vi "serpenbot_DDPG_control.vi"() -> ()   [LabVIEW 2019]
uses:
  <vilib>/Analysis/Matrix/Datatypes/RealMatrix.ctl
  <vilib>/Analysis/Matrix/NI_Matrix.lvlib
  <vilib>/Analysis/NI_AALBase.lvlib
  <vilib>/Analysis/baseanly.llb/Real A x B.vi
  <vilib>/Analysis/Matrix/Numeric/Conversions/Array To Matrix - RA.vi
  <vilib>/Analysis/Matrix/Numeric/Subtract/Subtract - RM,RM.vi
  <vilib>/Analysis/NI_AALPro.lvlib
  <vilib>/Analysis/_algsub.llb/Real PseudoInverse Matrix.vi
panel:
  out "error out Y":errorcluster
  out "error out X":errorcluster
  in  "goal y":dbl
  in  "goal x":dbl
  out "control_loop_time":u32
  in  "stop":bool
  in  "Logging":bool caption="Enable"
  out "laser control value":dbl[](array[numeric])
  in  "k":T1
  in  "Diode Current\nSetting":dbl=3.0
  in  "Laser Repetition\nFrequency":i32=50000
  in  "VISA resource name":refnum<visa-resource-name>="COM14"
  in  "baud rate (9600)":u32=9600
  out "error out":errorcluster
  out "Identification system 1":string
  out "Conn. axes system 1":string[](array[string])
  out "Identification system 2":string
  out "Conn. axes system  2":string[](array[string])
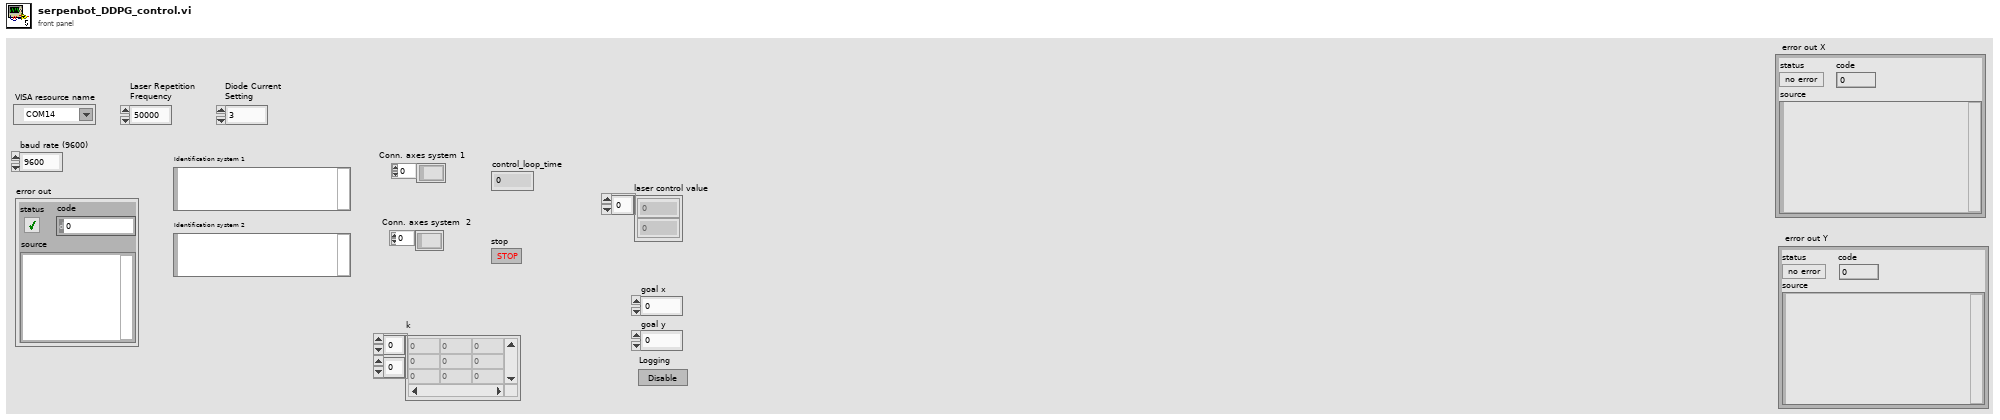
[diagram p1: front panel]
types:
  T1 = typedef "NI_Matrix.lvlib/RealMatrix.ctl" = dbl[][]
  T2 = cluster{"RS232 settings":cluster{"Portnumber":i32, "Baudrate":u16}, "USB settings":cluster{"S/N":string, "USB Search?":bool}, "TCP/IP settings":cluster{"Host address/name":string, "Port":i32, "Board":i32, "TCP/IP Search?":bool}}
  T3 = cluster{"Check FRF?":bool, "Referencing mode":enum16{"FRF (-> FNL)", "FRF", "FNL", "FPL", "RON OFF"}[]}
  T4 = cluster{"Force?":bool, "Dialog?":bool, "Stages":string[]}
  T5 = cluster{"Position":cluster{"x":sgl, "y":sgl}, "Angle":sgl, "Scale":sgl, "Score":sgl, "Bounding Box":cluster{"x":sgl, "y":sgl}[]}[]
  T6 = cluster{"[0]":cluster{"Position":cluster{"x":sgl, "y":sgl}, "Angle":sgl, "Scale":sgl, "Score":sgl, "Bounding Box":cluster{"x":sgl, "y":sgl}[]}, "[1]":cluster{"Position":cluster{"x":sgl, "y":sgl}, "Angle":sgl, "Scale":sgl, "Score":sgl, "Bounding Box":cluster{"x":sgl, "y":sgl}[]}, "[2]":cluster{"Position":cluster{"x":sgl, "y":sgl}, "Angle":sgl, "Scale":sgl, "Score":sgl, "Bounding Box":cluster{"x":sgl, "y":sgl}[]}, "[3]":cluster{"Position":cluster{"x":sgl, "y":sgl}, "Angle":sgl, "Scale":sgl, "Score":sgl, "Bounding Box":cluster{"x":sgl, "y":sgl}[]}, "[4]":cluster{"Position":cluster{"x":sgl, "y":sgl}, "Angle":sgl, "Scale":sgl, "Score":sgl, "Bounding Box":cluster{"x":sgl, "y":sgl}[]}, "[5]":cluster{"Position":cluster{"x":sgl, "y":sgl}, "Angle":sgl, "Scale":sgl, "Score":sgl, "Bounding Box":cluster{"x":sgl, "y":sgl}[]}, "[6]":cluster{"Position":cluster{"x":sgl, "y":sgl}, "Angle":sgl, "Scale":sgl, "Score":sgl, "Bounding Box":cluster{"x":sgl, "y":sgl}[]}, "[7]":cluster{"Position":cluster{"x":sgl, "y":sgl}, "Angle":sgl, "Scale":sgl, "Score":sgl, "Bounding Box":cluster{"x":sgl, "y":sgl}[]}, "[8]":cluster{"Position":cluster{"x":sgl, "y":sgl}, "Angle":sgl, "Scale":sgl, "Score":sgl, "Bounding Box":cluster{"x":sgl, "y":sgl}[]}}
  T7 = cluster{"Position":cluster{"x":sgl, "y":sgl}, "Angle":sgl, "Scale":sgl, "Score":sgl, "Bounding Box":cluster{"x":sgl, "y":sgl}[]}
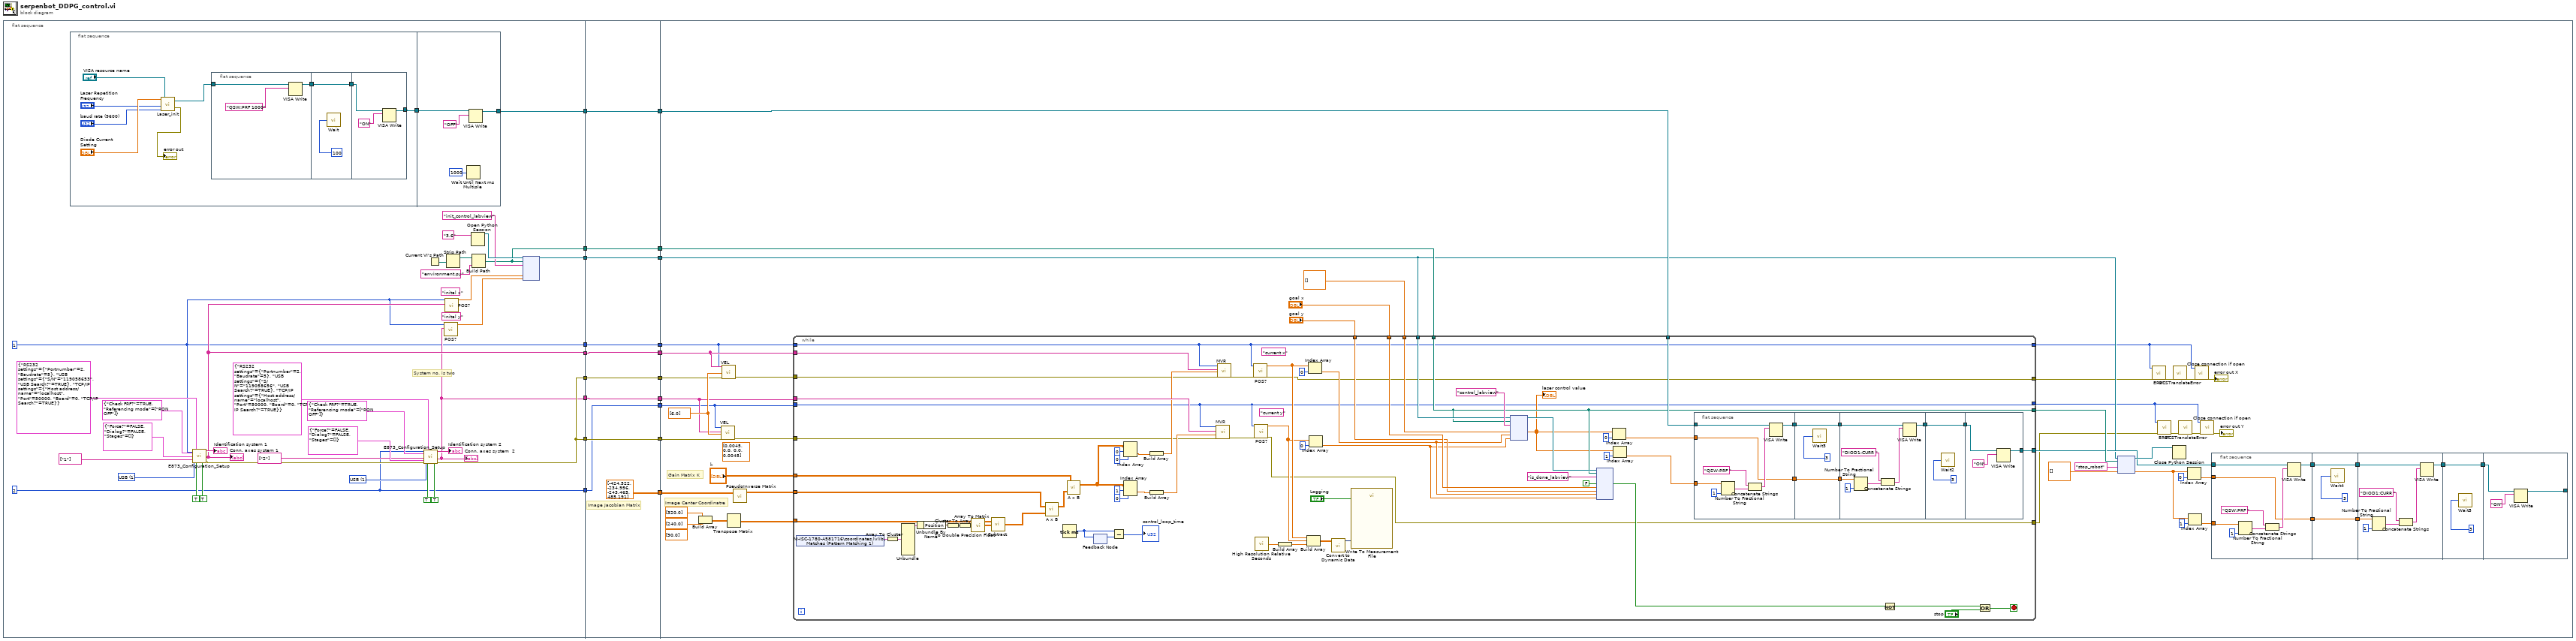
[diagram p0: block diagram]
diagram:
  n1 = flat-sequence {
    tunnel: [w52] -> w19
    tunnel: [w22] -> w18
    tunnel: [w24] -> w17
    tunnel: [w33] -> w16
    tunnel: [w23] -> w15
    tunnel: [w34] -> w14
    tunnel: [w33] -> w13
    tunnel: [w26] -> w12
    tunnel: [w25] -> w11
    tunnel: w19 -> [w84]
    tunnel: [w84] -> w10
    tunnel: w18 -> [w83]
    tunnel: w17 -> [w82]
    tunnel: w16 -> [w81]
    tunnel: w15 -> [w80]
    tunnel: w14 -> [w78]
    tunnel: [w83] -> w9
    tunnel: [w82] -> w8
    tunnel: [w81] -> w7
    tunnel: [w80] -> w6
    tunnel: w13 -> [w79]
    tunnel: [w79] -> w5
    tunnel: [w78] -> w4
    tunnel: [T1 [[-424.522, -234.956], [-243.465, 485.191]] ("J_init 2")] -> w3
    tunnel: w12 -> [w76]
    tunnel: w11 -> [w75]
    tunnel: [w76] -> w2
    tunnel: [w75] -> w1
    tunnel: w10 -> [w132]
    tunnel: w9 -> [w117]
    tunnel: w8 -> [w124]
    tunnel: w7 -> [w127]
    tunnel: w6 -> [w122]
    tunnel: w5 -> [w126]
    tunnel: w4 -> [w116]
    tunnel: w3 -> [w125]
    tunnel: w2 -> [w115]
    tunnel: w1 -> [w98]
    frame #0 {
      (unwired) "inital y"
      (unwired) "inital x"
      w37 = u16 1 items=["RS232", "USB", "TCP/IP"] ("Interface")
      w40 = u16 1 items=["RS232", "USB", "TCP/IP"] ("Interface")
      w34 = 2 ("System no.")
      w22 = 1 ("System no.")
      # "System no. is two"
      n2 = flat-sequence {
        tunnel: [w54] -> w53
        tunnel: w53 -> [w72]
        tunnel: [w71] -> w52
        frame #0 {
          n3 = call "Laser_init.vi"("baud rate (9600)"="baud rate (9600)", "Laser Repetition\nFrequency"="Laser Repetition\nFrequency", "VISA resource name"="VISA resource name", "Diode Current\nSetting"="Diode Current\nSetting") -> ("error out"=→"error out":errorcluster, "VISA Refnum out"=w55:refnum<visa-resource-name>)
          n4 = flat-sequence {
            tunnel: w55 -> [w65]
            tunnel: [w64] -> w62
            tunnel: w62 -> [w67]
            tunnel: [w67] -> w61
            tunnel: w61 -> [w68]
            tunnel: [w69] -> w54
            frame #0 {
              n5 = VISA Write(VISA resource name=w65, write buffer="QSW:PRF 1000" ("string")) -> (VISA resource name out=w64:refnum<visa-resource-name>)  [unwired: 1 in, 2 out]
            }
            frame #1 {
              n6 = call "Wait"("Count(mSec)"=u32 100) -> ()  [unwired: 1 out]
            }
            frame #2 {
              n7 = VISA Write(VISA resource name=w68, write buffer="ON") -> (VISA resource name out=w69:refnum<visa-resource-name>)  [unwired: 1 in, 2 out]
            }
          }
        }
        frame #1 {
          n8 = Wait Until Next ms Multiple(millisecond multiple=u32 1000) -> ()  [unwired: 1 out]
          n9 = VISA Write(VISA resource name=w72, write buffer="OFF") -> (VISA resource name out=w71:refnum<visa-resource-name>)  [unwired: 1 in, 2 out]
        }
      }
      n10 = call "E873_Configuration_Setup.vi"("System no."=w22, "Referencing"=T3 {"Check FRF?"=TRUE, "Referencing mode"=[enum."RON OFF"]}, "Interface"=w40, "All axes?"=TRUE, "Axes to move"=string[] ["1"], "Interface settings"=T2 {"RS232 settings"={"Portnumber"=2, "Baudrate"=5}, "USB settings"={"S/N"="119058653", "USB Search?"=TRUE}, "TCP/IP settings"={"Host address/name"="localhost", "Port"=50000, "Board"=0, "TCP/IP Search?"=TRUE}}, "Stage selection"=T4 {"Force?"=FALSE, "Dialog?"=FALSE, "Stages"=[]}, "Switch servo on?"=TRUE ("Use dialog to define\nconnected stages?")) -> ("Identification"=→"Identification system 1":string, "Conn. \nAxes"=w24:string[], "error out"=w49:errorcluster)  [unwired: 4 in, 5 out]
      "Conn. axes system 1" <- w24
      n11 = call "E873_Configuration_Setup.vi"("System no."=w34, "Referencing"=T3 {"Check FRF?"=TRUE, "Referencing mode"=[enum."RON OFF"]}, "Interface"=w37, "All axes?"=TRUE, "Axes to move"=string[] ["2"], "error in"=w49, "Interface settings"=T2 {"RS232 settings"={"Portnumber"=2, "Baudrate"=5}, "USB settings"={"S/N"="119058656", "USB Search?"=TRUE}, "TCP/IP settings"={"Host address/name"="localhost", "Port"=50000, "Board"=0, "TCP/IP Search?"=TRUE}}, "Stage selection"=T4 {"Force?"=FALSE, "Dialog?"=FALSE, "Stages"=[]}, "Switch servo on?"=TRUE ("Use dialog to define\nconnected stages?")) -> ("Identification"=→"Identification system 2":string, "Conn. \nAxes"=w23:string[], "error out"=w33:errorcluster)  [unwired: 3 in, 5 out]
      "Conn. axes system  2" <- w23
      n12 = Current VI's Path() -> (path=w32:path)
      n13 = call "POS?.vi"("System no."=w22, "Axes to query"=w23) -> ("Position"=w20:dbl[])  [unwired: 3 in, 14 out]
      n14 = call "POS?.vi"("System no."=w22, "Axes to query"=w24) -> ("Position"=w21:dbl[])  [unwired: 3 in, 14 out]
      n15 = Strip Path(path=w32) -> (stripped path=w31:path)  [unwired: 1 out]
      n16 = Open Python Session(python version="3.6" ("Python version")) -> (session out=w28:refnum<k35>)  [unwired: 2 in, 1 out]
      n17 = Build Path(base path=w31, name or relative path="environment.py") -> (appended path=w26:path)
      n18 = node(w28, w26, "init_control_labview" ("function name"), w21, w20) -> (w25:refnum<k35>)  [unwired: 5 in, 3 out]
    }
    frame #1 {
      # "Image Jacobian Matrix"
    }
    frame #2 {
      w128 = dbl[] [6.0] ("Velocity values")
      (unwired) T1 [[0.0045, 0.0], [0.0, 0.0045]] ("J_init 2")
      (unwired) dbl[] [90.0] ("element")
      # "Gain Matrix K"
      # "Image Center Coordinatre"
      n19 = Build Array(dbl[] [320.0] ("element"), dbl[] [240.0] ("element")) -> (w129:T1)
      n20 = call "VEL.vi"("System no."=w116, "Axes to set"=w122, "Velocity values"=w128, "error in"=w126) -> ("error out"=w121:errorcluster)  [unwired: 2 in, 13 out]
      n21 = call "VEL.vi"("System no."=w117, "Axes to set"=w124, "Velocity values"=w128, "error in"=w127) -> ("error out"=w123:errorcluster)  [unwired: 2 in, 13 out]
      n22 = Transpose Matrix(1:w129) -> (0:w118:T1)
      n23 = call-poly <vilib>:"PseudoInverse Matrix.vi"("Input Matrix"=w125) -> ("PseudoInverse Matrix"=w119:T1)  [unwired: 1 in, 1 out]
      n24 = while {
        tunnel: w121 -> [w185]
        tunnel: w116 -> [w134]
        tunnel: w122 -> [w203]
        tunnel: w123 -> [w186]
        tunnel: w124 -> [w202]
        tunnel: w117 -> [w136]
        tunnel: w119 -> [w191]
        tunnel: "k" -> [w190]
        tunnel: w118 -> [w189]
        tunnel: w132 -> [w164]
        tunnel: w115 -> [w151]
        tunnel: w98 -> [w159]
        tunnel: dbl[] [] -> [w158]
        tunnel: "goal x" -> [w157]
        tunnel: "goal y" -> [w156]
        tunnel: [w151] -> w105
        tunnel: [w150] -> w104
        tunnel: [w136] -> w87
        tunnel: [w135] -> w88
        tunnel: [w134] -> w86
        tunnel: [w133] -> w85
        stop <- w168 stop-if-true
        (unwired) "current y"
        (unwired) "current x"
        n25 = shared-variable "NI-ISC-1780-A581716\\coordinates.lvlib\\Matches (Pattern Matching 1)"() -> (w178:T5)  [unwired: 1 in, 1 out]
        n26 = Array To Cluster(array=w178) -> (cluster=w179:T6)
        n27 = Unbundle(w179) -> ("[0]"=w180:T7)  [unwired: 8 out]
        n28 = Unbundle By Name(w180) -> ("Position"=w181:cluster{"x":sgl, "y":sgl})
        n29 = Cluster To Array(cluster=w181) -> (array=w182:sgl[])
        n30 = To Double Precision Float(number=w182) -> (double precision float=w183:dbl[])
        n31 = call-poly <vilib>:"Array To Matrix.vi"("Real 1D Array"=w183) -> ("Real Matrix (Column Vector)"=w177:T1)
        n32 = call-poly <vilib>:"Subtract.vi"("Real Matrix B"=w177, "Real Matrix A"=w189) -> ("A - B"=w197:T1)
        n33 = call-poly <vilib>:"A x B.vi"("B"=w197, "A"=w191) -> ("A x B"=w195:T1)  [unwired: 1 out]
        n34 = Tick Count (ms)() -> (millisecond timer value=w167:u32)
        n35 = call-poly <vilib>:"A x B.vi"("B"=w195, "A"=w190) -> ("A x B"=w196:T1)  [unwired: 1 out]
        n36 = feedback #1() -> (w192:u32)  [unwired: 1 in]
        n37 = feedback-in #1(w167) -> ()
        n38 = Subtract(x=w167, y=w192) -> (x-y=→"control_loop_time":u32)
        n39 = Index Array(array=w196, index (row)=0, index (col)=0) -> (element=w188:dbl)
        n40 = Index Array(array=w196, index (row)=1, index (col)=0) -> (element=w187:dbl)
        n41 = Build Array(w188) -> (w194:dbl[])
        n42 = Build Array(w187) -> (w193:dbl[])
        n43 = call "MVR.vi"("System no."=w134, "Axes to move"=w203, "Position values"=w193, "error in"=w185) -> ("error out"=w170:errorcluster)  [unwired: 1 in, 14 out]
        n44 = call "MVR.vi"("System no."=w136, "Axes to move"=w202, "Position values"=w194, "error in"=w186) -> ("error out"=w171:errorcluster)  [unwired: 1 in, 14 out]
        n45 = call "POS?.vi"("System no."=w136, "error in"=w171) -> ("Position"=w149:dbl[], "error out"=w135:errorcluster)  [unwired: 3 in, 13 out]
        n46 = call "POS?.vi"("System no."=w134, "error in"=w170) -> ("Position"=w147:dbl[], "error out"=w133:errorcluster)  [unwired: 3 in, 13 out]
        n47 = call <vilib>:"High Resolution Relative Seconds.vi"() -> ("relative seconds"=w173:dbl)
        n48 = Build Array(w173) -> (w172:dbl[])
        n49 = Build Array(w149, w147, w172) -> (w175:dbl[][])
        n50 = Index Array(array=w149, index=0) -> (element=w138:dbl)
        n51 = Index Array(array=w147, index=0) -> (element=w137:dbl)
        n52 = call "Convert to Dynamic Data"("2D Array"=w175) -> ("Dynamic Data Type"=w174:dynamicdata)  [unwired: 3 in]
        n53 = call "Write To Measurement File"("Signals"=w174, "Enable"="Logging") -> ()  [unwired: 15 in, 3 out]
        n54 = node(w159, w151, "control_labview" ("function name"), w158, w138, w137) -> (w162:refnum<k35>, w142:dbl[])  [unwired: 3 in, 3 out]
        "laser control value" <- w142
        n55 = node(w162, w151, "is_done_labview" ("function name"), FALSE, w157, w156, w138, w137) -> (w139:bool)  [unwired: 5 in, 4 out]
        n56 = Index Array(array=w142, index=0) -> (element=w145:dbl)
        n57 = Index Array(array=w142, index=1) -> (element=w141:dbl)
        n58 = flat-sequence {
          tunnel: w164 -> [w207]
          tunnel: [w206] -> w153
          tunnel: w141 -> [w205]
          tunnel: w145 -> [w204]
          tunnel: [w204] -> w152
          tunnel: [w214] -> w155
          tunnel: [w212] -> w154
          tunnel: w153 -> [w214]
          tunnel: w152 -> [w212]
          tunnel: [w221] -> w166
          tunnel: w155 -> [w219]
          tunnel: w154 -> [w216]
          tunnel: w166 -> [w223]
          tunnel: [w223] -> w165
          tunnel: w165 -> [w225]
          tunnel: [w224] -> w150
          frame #0 {
            n59 = Number To Fractional String(number=w205, precision (6)=i16 1) -> (F-format string=w210:string)  [unwired: 2 in]
            n60 = Concatenate Strings("QSW:PRF " ("string"), w210) -> (w211:string)
            n61 = VISA Write(VISA resource name=w207, write buffer=w211) -> (VISA resource name out=w206:refnum<visa-resource-name>)  [unwired: 1 in, 2 out]
          }
          frame #1 {
            n62 = call "Wait3"("Count(mSec)"=u32 3) -> ()  [unwired: 1 out]
          }
          frame #2 {
            n63 = Number To Fractional String(number=w216, precision (6)=i16 1) -> (F-format string=w217:string)  [unwired: 2 in]
            n64 = Concatenate Strings("DIOD1:CURR " ("string"), w217) -> (w220:string)
            n65 = VISA Write(VISA resource name=w219, write buffer=w220) -> (VISA resource name out=w221:refnum<visa-resource-name>)  [unwired: 1 in, 2 out]
          }
          frame #3 {
            n66 = call "Wait2"("Count(mSec)"=u32 3) -> ()  [unwired: 1 out]
          }
          frame #4 {
            n67 = VISA Write(VISA resource name=w225, write buffer="ON") -> (VISA resource name out=w224:refnum<visa-resource-name>)  [unwired: 1 in, 2 out]
          }
        }
        n68 = Not(x=w139) -> (.not. x?=w140:bool)
        n69 = Or(x=w140, y="stop") -> (x .or. y?=w168:bool)
      }
      n70 = node(w98, w105, "stop_robot" ("function name"), dbl[] []) -> (w106:refnum<k35>, w99:dbl[])  [unwired: 1 in, 3 out]
      n71 = call "ERR?.vi"("System no."=w87, "error in"=w88) -> ("error out"=w92:errorcluster)  [unwired: 17 out]
      n72 = call "ERR?.vi"("System no."=w86, "error in"=w85) -> ("error out"=w89:errorcluster)  [unwired: 17 out]
      n73 = Close Python Session(session in=w106) -> ()  [unwired: 1 in, 1 out]
      n74 = call "GCSTranslateError.vi"("error in"=w92) -> ("error out"=w93:errorcluster)  [unwired: 18 out]
      n75 = call "GCSTranslateError.vi"("error in"=w89) -> ("error out"=w90:errorcluster)  [unwired: 18 out]
      n76 = Index Array(array=w99, index=0) -> (element=w101:dbl)
      n77 = Index Array(array=w99, index=1) -> (element=w100:dbl)
      n78 = call "Close connection if open.vi"("System no."=w87, "error in"=w93) -> ("error out"=→"error out X":errorcluster)  [unwired: 1 in, 16 out]
      n79 = call "Close connection if open.vi"("System no."=w86, "error in"=w90) -> ("error out"=→"error out Y":errorcluster)  [unwired: 1 in, 16 out]
      n80 = flat-sequence {
        tunnel: w104 -> [w230]
        tunnel: [w229] -> w114
        tunnel: w100 -> [w228]
        tunnel: w101 -> [w227]
        tunnel: [w227] -> w113
        tunnel: [w237] -> w112
        tunnel: [w235] -> w111
        tunnel: w114 -> [w237]
        tunnel: w113 -> [w235]
        tunnel: [w244] -> w110
        tunnel: w112 -> [w242]
        tunnel: w111 -> [w239]
        tunnel: w110 -> [w246]
        tunnel: [w246] -> w109
        tunnel: w109 -> [w248]
        tunnel: [w247] -> _
        frame #0 {
          n81 = Number To Fractional String(number=w228, precision (6)=i16 1) -> (F-format string=w233:string)  [unwired: 2 in]
          n82 = Concatenate Strings("QSW:PRF " ("string"), w233) -> (w234:string)
          n83 = VISA Write(VISA resource name=w230, write buffer=w234) -> (VISA resource name out=w229:refnum<visa-resource-name>)  [unwired: 1 in, 2 out]
        }
        frame #1 {
          n84 = call "Wait4"("Count(mSec)"=u32 3) -> ()  [unwired: 1 out]
        }
        frame #2 {
          n85 = Number To Fractional String(number=w239, precision (6)=i16 1) -> (F-format string=w240:string)  [unwired: 2 in]
          n86 = Concatenate Strings("DIOD1:CURR " ("string"), w240) -> (w243:string)
          n87 = VISA Write(VISA resource name=w242, write buffer=w243) -> (VISA resource name out=w244:refnum<visa-resource-name>)  [unwired: 1 in, 2 out]
        }
        frame #3 {
          n88 = call "Wait5"("Count(mSec)"=u32 3) -> ()  [unwired: 1 out]
        }
        frame #4 {
          n89 = VISA Write(VISA resource name=w248, write buffer="ON") -> (VISA resource name out=w247:refnum<visa-resource-name>)  [unwired: 1 in, 2 out]
        }
      }
    }
  }
